vi "BAR0469_MainProject2.vi"() -> ()   [LabVIEW 2021]
panel:
  out "Vypoctena Fmez":dbl caption="Vypoctena Fmez (Hz)"
  out "Aktuální amplituda (V)":dbl
  out "A/f charakteristika":cluster{dbl[], dbl[]}(graph)
  in  "liner/log":bool
  in  "Typ filtru":string
  in  "Krok":dbl min=0.0 max=10000.0
  in  "Aproximace":string
  in  "Amplituda (V)":dbl min=0.0 max=10.0
  out "Aktuální frekvence (Hz)":dbl
  in  "volt/dB":bool
  in  "Vysoká frekvence (Hz)":dbl min=0.0 max=10000.0
  in  "Nízká frekvence (Hz)":dbl min=0.0 max=10000.0
  in  "Øád":i8 min=0 max=6
  in  "fmin (Hz)":dbl min=0.0 max=10000.0
  in  "fmax (Hz)":dbl min=0.0 max=1000.0
  in  "Username":string caption="Jméno Uživatele"
  in  "Stop":bool caption="OK Button"
  in  "Save button":bool caption="OK Button"
  in  "Load":bool caption="OK Button"
  in  "Reincialization Button":bool caption="OK Button"
  in  "Start Button":bool caption="OK Button"
  out "Datum a èas mìøení":string
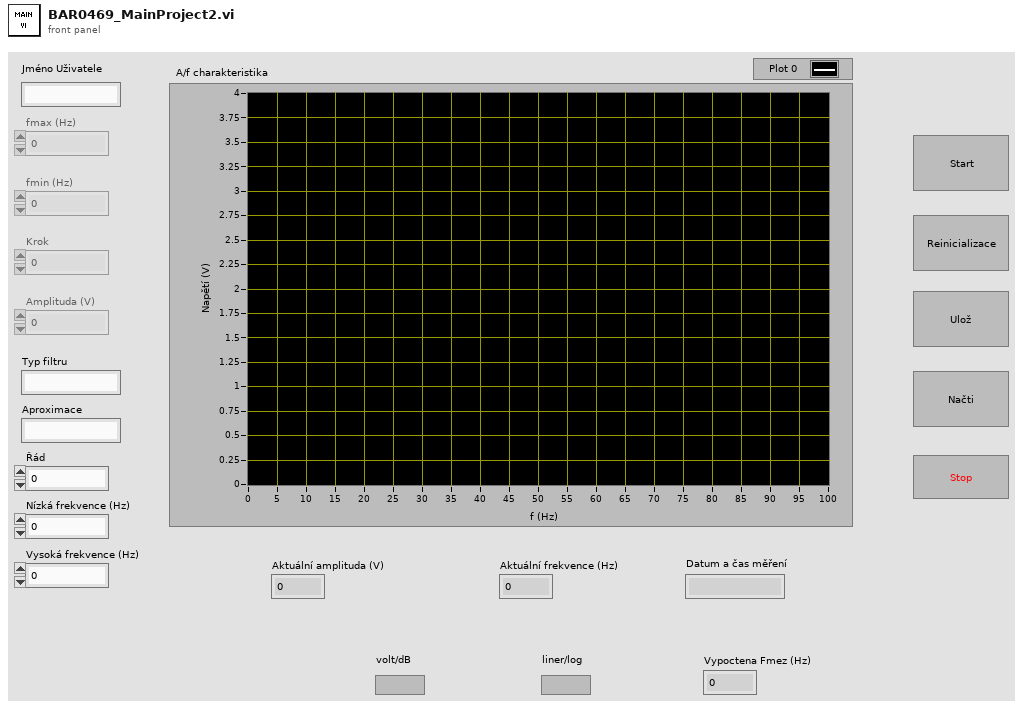
[diagram p1: front panel]
types:
  T1 = enum8{"Enabled", "Disabled", "Disabled and Grayed Out"}
  T2 = cluster{"Frequency (Hz)":dbl[], "Pøenos (dB)":dbl[]}
  T3 = cluster{"Frequency (Hz)":dbl[], "Amplitude (V)":dbl[]}
  T4 = cluster{"String from file":string, "String from file":string, "String from file":string, "String from file":string, "String from file":string, "String from file":string, "String from file":string, "String from file":string, "String from file":string, "String from file":string, "String from file":string}
  T5 = cluster{"Frequency (Hz)":dbl[], "Amplitude (V)":dbl[], "Pøenos (dB)":dbl[]}
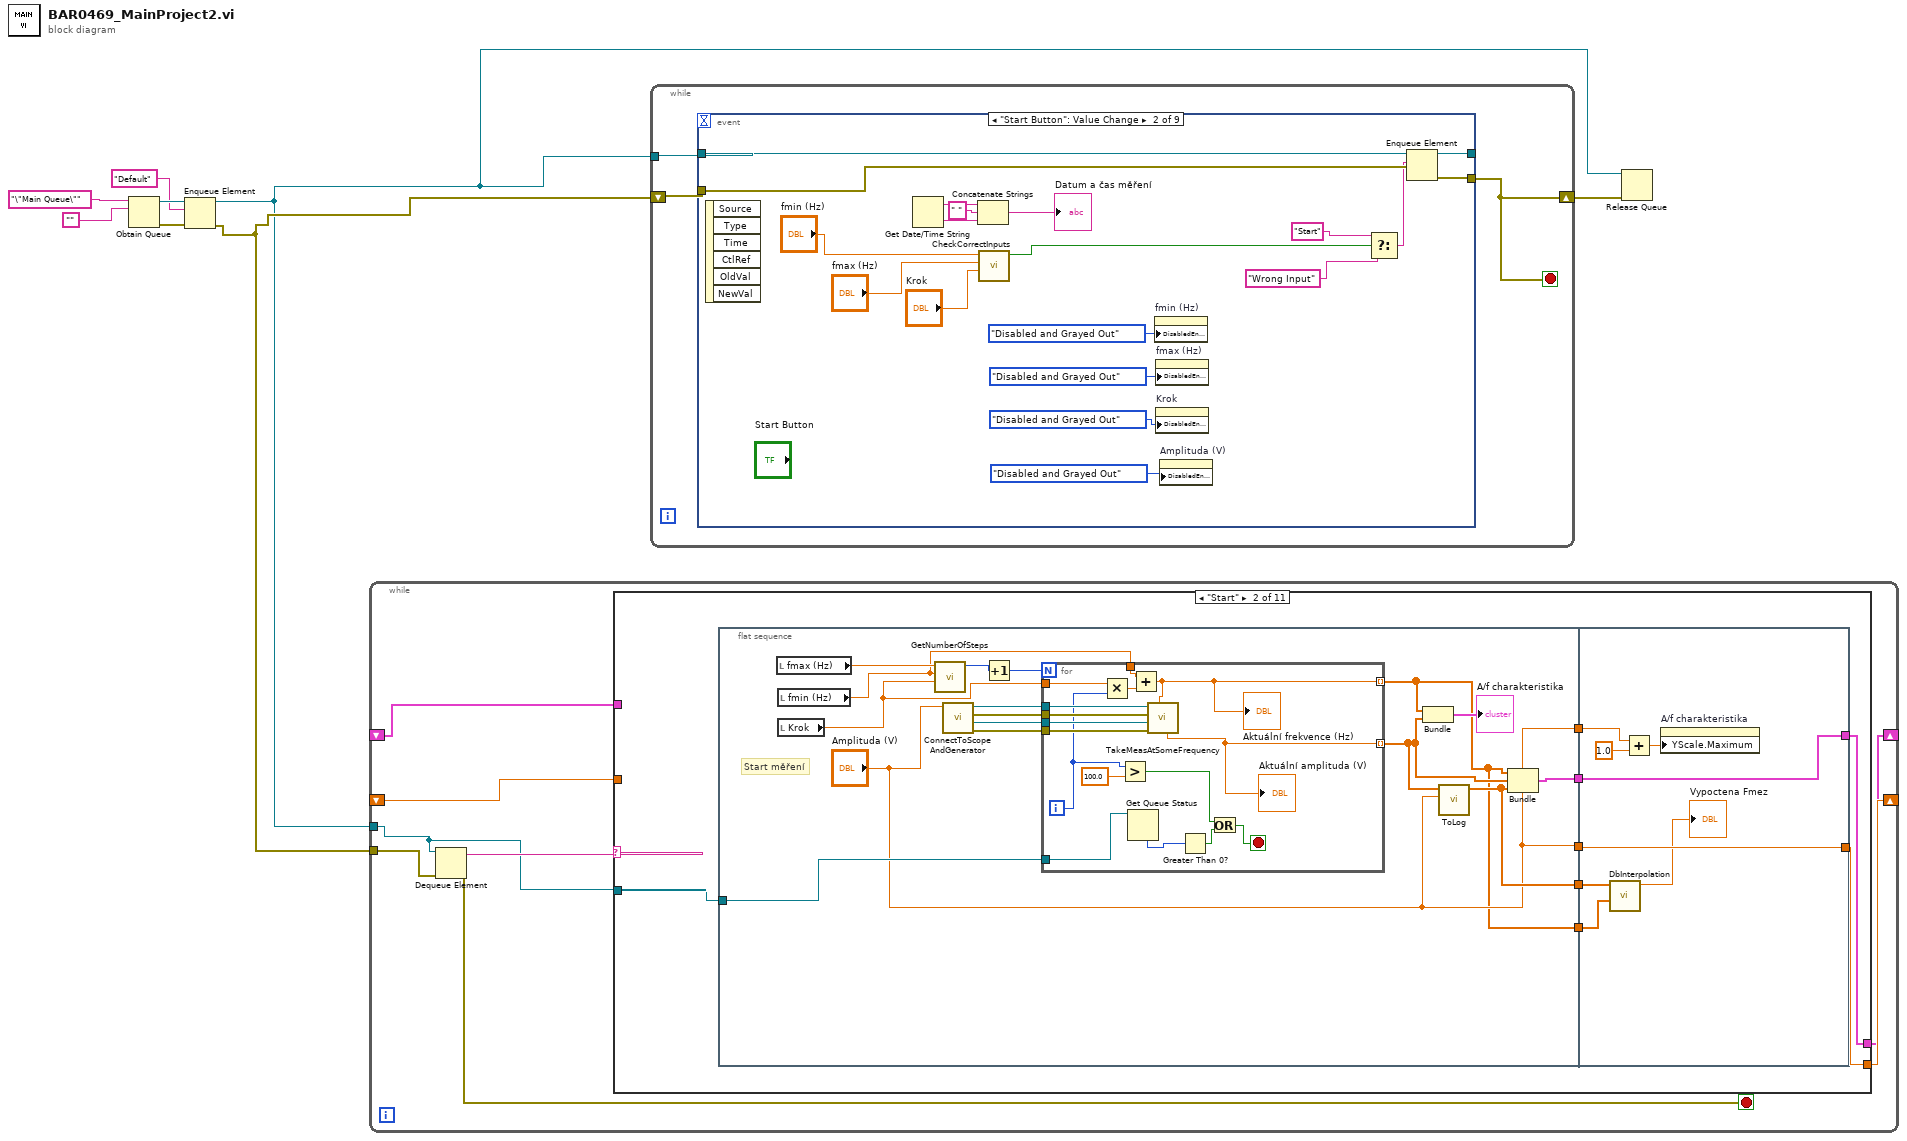
[diagram p0: block diagram]
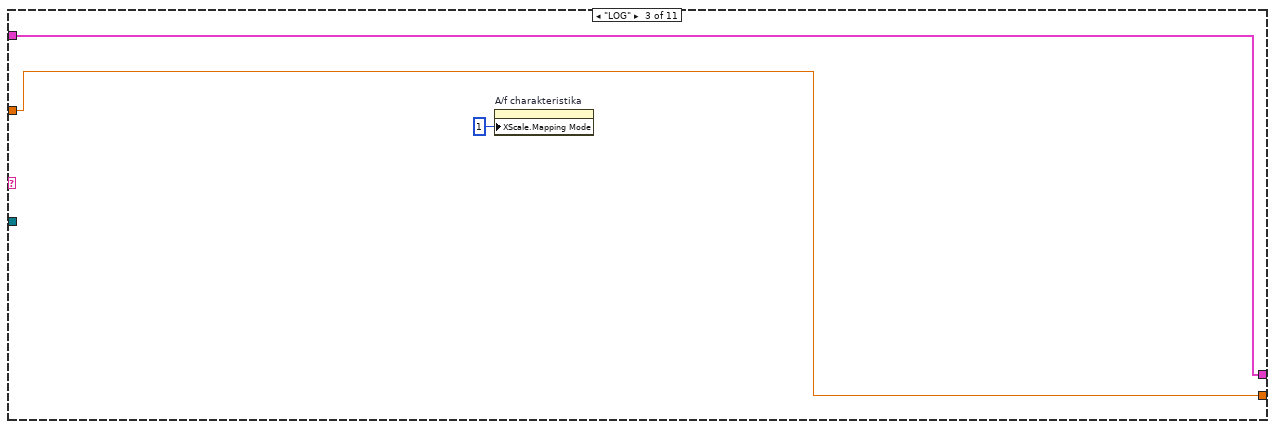
[diagram p3: hidden frame]
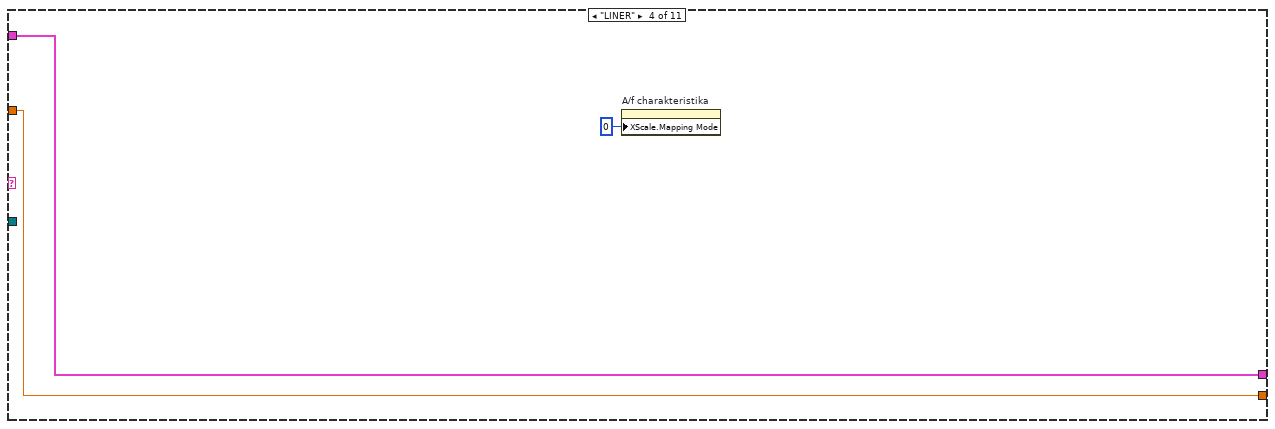
[diagram p4: hidden frame]
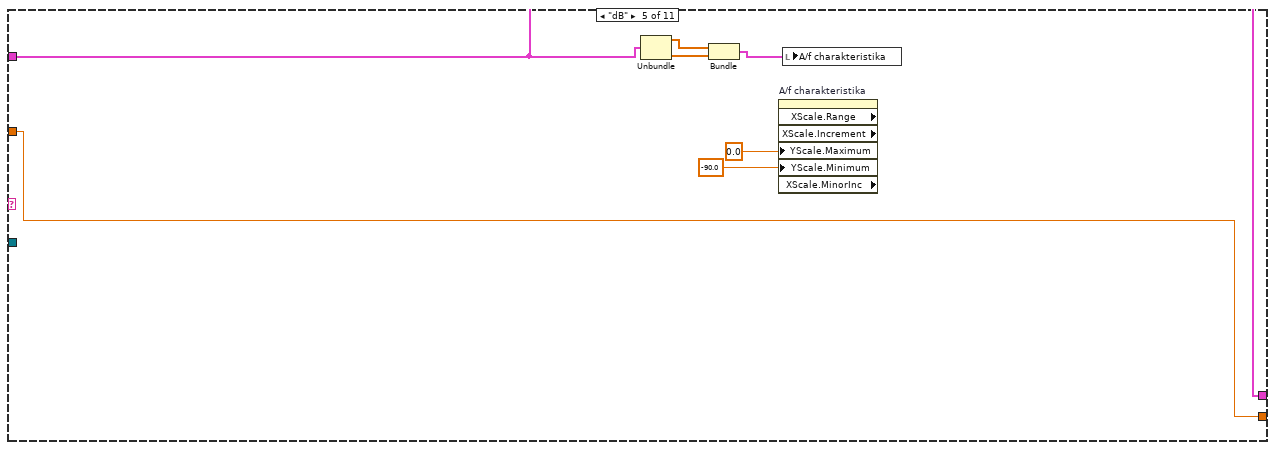
[diagram p5: hidden frame]
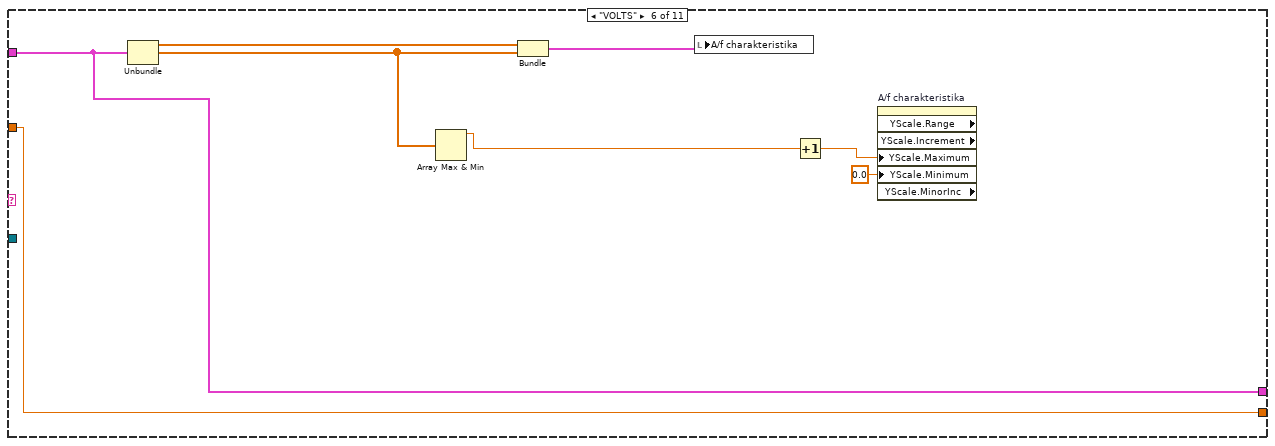
[diagram p6: hidden frame]
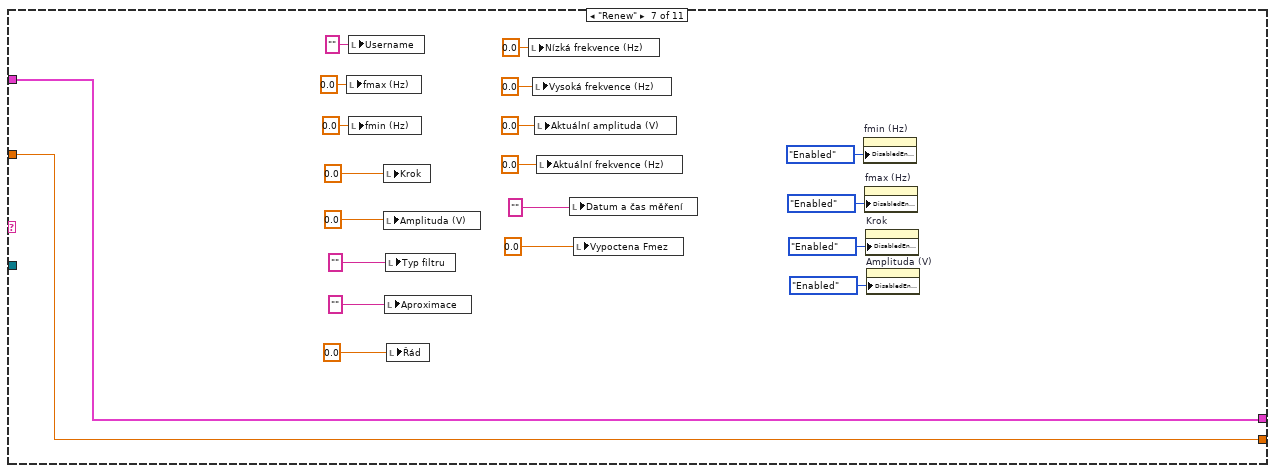
[diagram p7: hidden frame]
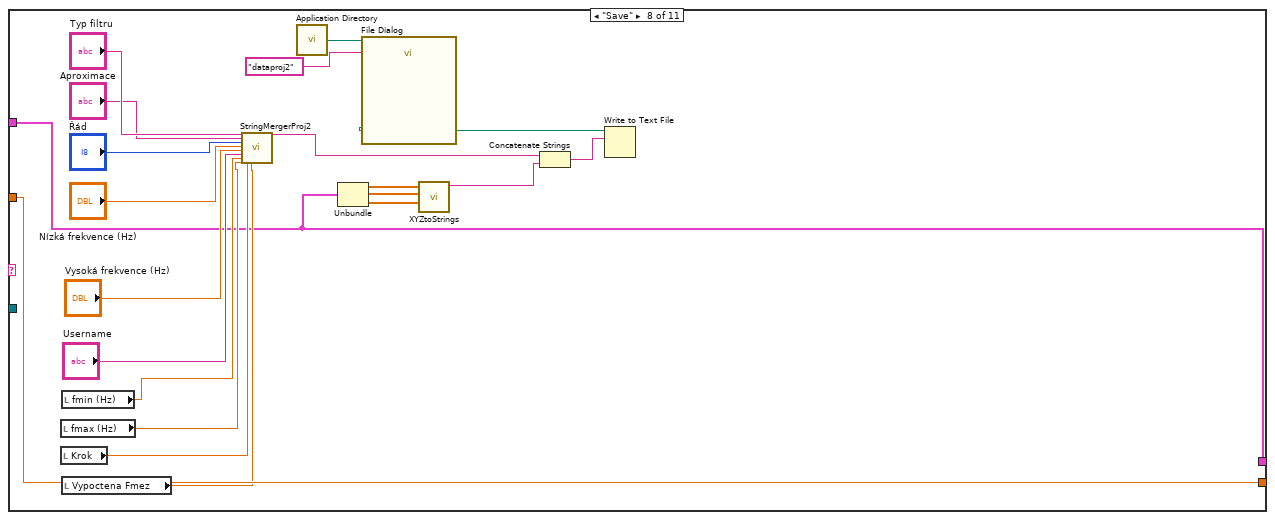
[diagram p8: hidden frame]
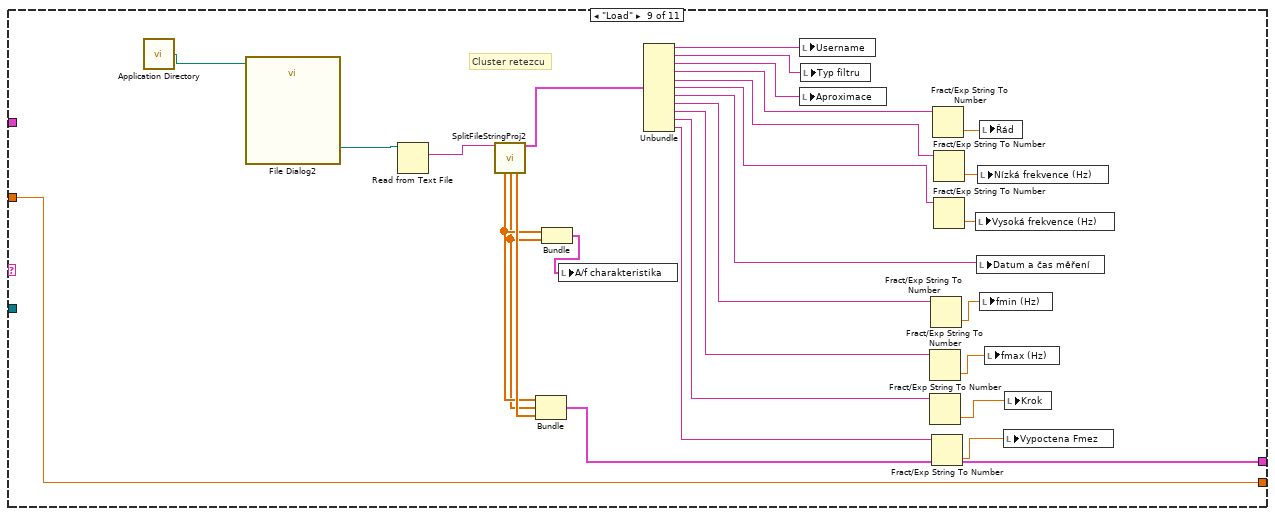
[diagram p9: hidden frame]
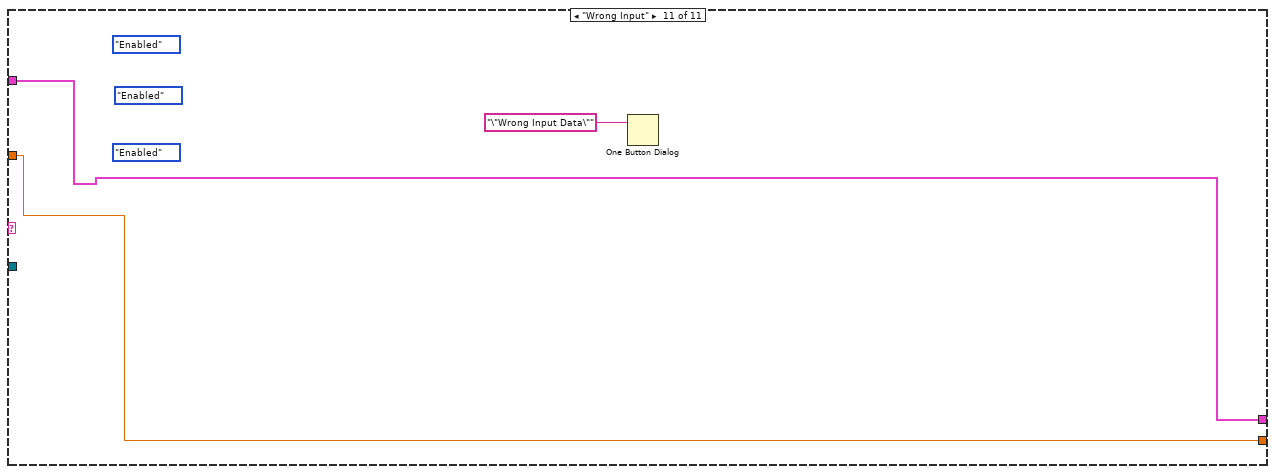
[diagram p11: hidden frame]
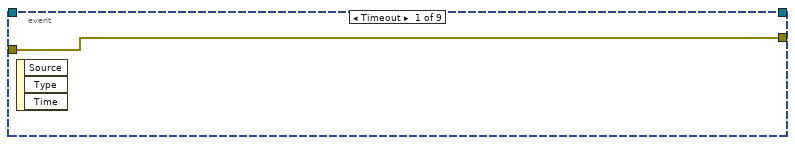
[diagram p12: hidden frame]
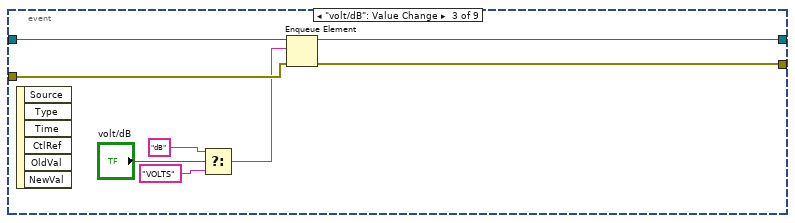
[diagram p13: hidden frame]
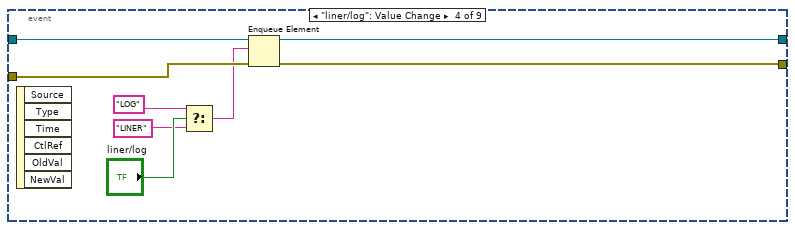
[diagram p14: hidden frame]
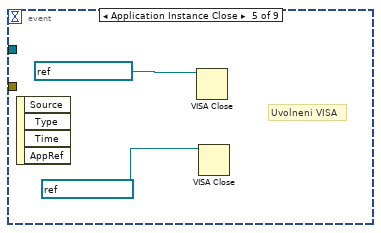
[diagram p15: hidden frame]
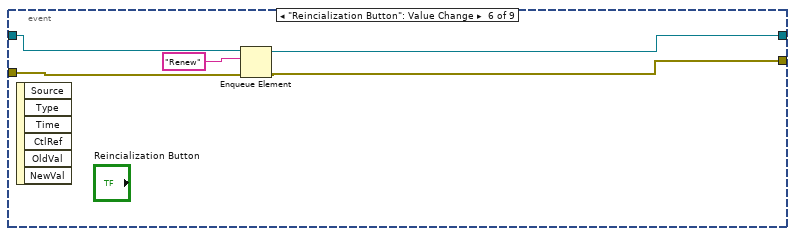
[diagram p16: hidden frame]
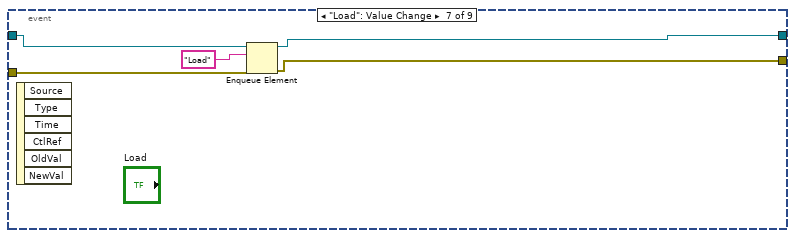
[diagram p17: hidden frame]
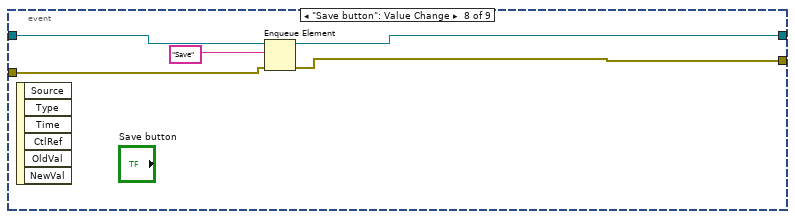
[diagram p18: hidden frame]
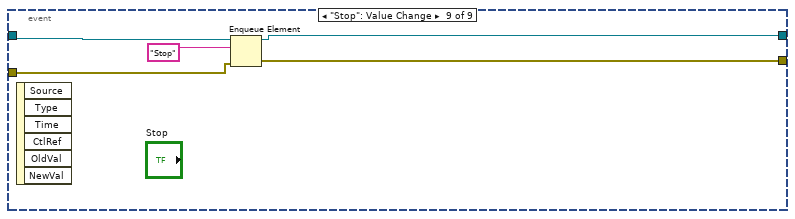
[diagram p19: hidden frame]
diagram:
  n1 = Obtain Queue(name (unnamed)="\"Main Queue\"", element data type="") -> (queue out=w6:refnum<queue>, error out=w5:errorcluster)  [unwired: 3 in, 1 out]
  n2 = Enqueue Element(queue=w6, element="Default", error in (no error)=w5) -> (queue out=w3:refnum<queue>, error out=w4:errorcluster)  [unwired: 1 in, 1 out]
  n3 = while {
    tunnel: w3 -> [w13]
    tunnel: w4 -> [w16]
    shift-right: [w12] -> _
    shift-left: _ -> [w11]
    shift-right: [w10] -> _
    shift-left: _ -> [w9]
    stop <- w15 stop-if-true
    n4 = Dequeue Element(queue=w13, error in (no error)=w16) -> (element=w14:string, error out=w15:errorcluster)  [unwired: 1 in, 2 out]
    n5 = case shown="\"Start\"" w14 {
      tunnel: w13 -> [_ w26 _ _ _ _ _ _ _ _ _]
      tunnel: [w18 w23 w67 w71 w77 w80 w107 w128 w156 w158 w160] -> w12
      tunnel: w11 -> [w18 _ w67 w71 w77 w80 w107 w128 w156 w158 w160]
      tunnel: [w17 w22 w68 w72 w73 w83 w106 w114 w132 w157 w159] -> w10
      tunnel: w9 -> [w17 _ w68 w72 w73 w83 w106 w114 _ w157 w159]
      frame "Default", Default {
      }
      frame "Start" {
        n6 = flat-sequence {
          tunnel: w26 -> [w35]
          tunnel: ["Amplituda (V)"] -> w25
          tunnel: ["Amplituda (V)"] -> w24
          tunnel: [w32] -> w21
          tunnel: [w31] -> w20
          tunnel: [w29] -> w19
          tunnel: w25 -> [w64]
          tunnel: w24 -> [w63]
          tunnel: [w63] -> w23
          tunnel: [w62] -> w22
          tunnel: w21 -> [w62]
          tunnel: w20 -> [w61]
          tunnel: w19 -> [w60]
          frame #0 {
            # "Start mìøení"
            n7 = local read "fmax (Hz)"() -> (w38:dbl)
            n8 = local read "fmin (Hz)"() -> (w36:dbl)
            n9 = local read "Krok"() -> (w37:dbl)
            n10 = call "GetNumberOfSteps.vi"("Step"=w37, "Min"=w36, "Max"=w38) -> ("unsigned 64bit integer"=w28:u64)  [unwired: 8 in]
            n11 = call "ConnectToScopeAndGenerator.vi"("Input Number"="Amplituda (V)") -> ("GEN error out"=w39:errorcluster, "GEN resource output"=w40:refnum<visa-resource-name>, "OSC error out"=w41:errorcluster, "OSC Reference"=w42:refnum<visa-resource-name>)  [unwired: 7 in]
            n12 = Increment(x=w28) -> (x+1=w27:u64)
            n13 = for {
              N: w27 -> [_]
              tunnel: w42 -> [w58]
              tunnel: w41 -> [w57]
              tunnel: w40 -> [w56]
              tunnel: w39 -> [w55]
              tunnel: [w54] -> w33 mode=indexing
              tunnel: w37 -> [w53]
              tunnel: w36 -> [w51]
              tunnel: [w48] -> w29 mode=indexing
              tunnel: w35 -> [w49]
              i -> [w46]
              stop <- w44 stop-if-true
              n14 = Multiply(x=w53, y=w46) -> (x*y=w52:dbl)
              n15 = Greater?(x=w46, y=100.0) -> (0:w43:bool)
              n16 = Get Queue Status(queue=w49) -> (# elements in queue=w50:i32)  [unwired: 2 in, 7 out]
              n17 = Add(x=w51, y=w52) -> (x+y=w48:dbl)
              "Aktuální frekvence (Hz)" <- w48
              n18 = call "TakeMeasAtSomeFrequency.vi"("Generator Frequency"=w48, "GEN error"=w55, "GEN VISA"=w56, "Scope Error"=w57, "Scope VISA"=w58) -> ("max value"=w54:dbl)  [unwired: 1 in, 5 out]
              "Aktuální amplituda (V)" <- w54
              n19 = Greater Than 0?(x=w50) -> (x > 0?=w45:bool)
              n20 = Or(x=w43, y=w45) -> (x .or. y?=w44:bool)
            }
            n21 = Bundle(w29, w33) -> (→"A/f charakteristika":cluster{dbl[], dbl[]})  [unwired: 1 in]
            n22 = call "ToLog.vi"("Amplituda"="Amplituda (V)", "Pole vystupniho napeti"=w33) -> ("Napeti log"=w31:dbl[])  [unwired: 9 in]
            n23 = Bundle(w29, w33, "Napeti log"=w31) -> (w32:cluster{dbl[], dbl[], "Napeti log":dbl[]})  [unwired: 1 in]
          }
          frame #1 {
            n24 = call "DbInterpolation.vi"("Frequency"=w60, "Transfers"=w61) -> ("interpolated val"=→"Vypoctena Fmez":dbl)  [unwired: 9 in]
            n25 = Add(x=w64, y=1.0) -> (x+y=w66:dbl)
            n26 = property on="A/f charakteristika" class="XYGraph (strict)"("YScale.Maximum"=w66) -> ()  [unwired: 2 in, 2 out]
          }
        }
      }
      frame "LOG" {
        n27 = property on="A/f charakteristika" class="XYGraph (strict)"("XScale.Mapping Mode"=u8 1 ("X Scale.Mapping Mode")) -> ()  [unwired: 2 in, 2 out]
      }
      frame "LINER" {
        n28 = property on="A/f charakteristika" class="XYGraph (strict)"("XScale.Mapping Mode"=u8 0 ("Y Scale.Mapping Mode")) -> ()  [unwired: 2 in, 2 out]
      }
      frame "dB" {
        n29 = Unbundle(w73) -> ("Frequency (Hz)"=w76:dbl[], "Pøenos (dB)"=w75:dbl[])  [unwired: 1 out]
        n30 = Bundle("Frequency (Hz)"=w76, "Pøenos (dB)"=w75) -> (w74:T2)  [unwired: 1 in]
        n31 = property on="A/f charakteristika" class="XYGraph (strict)" props=["XScale", "Range", "XScale", "Increment", "YScale", "Maximum", "YScale", "Minimum", "XScale", "MinorInc"]("YScale.Maximum"=0.0 ("X Scale.Range:Maximum"), "YScale.Minimum"=-90.0 ("X Scale.Range:Minimum")) -> ()  [unwired: 2 in, 5 out]
        n32 = local write "A/f charakteristika"(w74) -> ()
      }
      frame "VOLTS" {
        n33 = Unbundle(w83) -> ("Frequency (Hz)"=w85:dbl[], "Amplitude (V)"=w82:dbl[])  [unwired: 1 out]
        n34 = Array Max & Min(array=w82) -> (max value=w81:dbl)  [unwired: 3 out]
        n35 = Bundle("Frequency (Hz)"=w85, "Amplitude (V)"=w82) -> (w84:T3)  [unwired: 1 in]
        n36 = local write "A/f charakteristika"(w84) -> ()
        n37 = Increment(x=w81) -> (x+1=w86:dbl)
        n38 = property on="A/f charakteristika" class="XYGraph (strict)" props=["YScale", "Range", "YScale", "Increment", "YScale", "Maximum", "YScale", "Minimum", "YScale", "MinorInc"]("YScale.Maximum"=w86, "YScale.Minimum"=0.0 ("Y Scale.Range:Minimum")) -> ()  [unwired: 2 in, 5 out]
      }
      frame "Renew" {
        n39 = local write "fmax (Hz)"(0.0 ("fmax (Hz)")) -> ()
        n40 = local write "Username"("" ("Username")) -> ()
        n41 = local write "fmin (Hz)"(0.0 ("fmin (Hz)")) -> ()
        n42 = local write "Krok"(0.0 ("Krok")) -> ()
        n43 = local write "Amplituda (V)"(0.0 ("Amplituda (V)")) -> ()
        n44 = local write "Aproximace"("" ("Aproximace")) -> ()
        n45 = local write "Typ filtru"("" ("Typ filtru")) -> ()
        n46 = local write "Øád"(0.0 ("Øád")) -> ()
        n47 = local write "Nízká frekvence (Hz)"(0.0 ("Nízká frekvence (Hz)")) -> ()
        n48 = local write "Vysoká frekvence (Hz)"(0.0 ("Vysoká frekvence (Hz)")) -> ()
        n49 = local write "Aktuální amplituda (V)"(0.0 ("Aktuální amplituda (V)")) -> ()
        n50 = local write "Aktuální frekvence (Hz)"(0.0 ("Aktuální frekvence (Hz)")) -> ()
        n51 = local write "Datum a èas mìøení"("" ("Datum a èas mìøení")) -> ()
        n52 = local write "Vypoctena Fmez"(0.0 ("Vypoctena Fmez")) -> ()
        n53 = property on="fmin (Hz)" class="DigNum (strict)"("DisabledEnum"=T1."Enabled" ("Disabled")) -> ()  [unwired: 2 in, 2 out]
        n54 = property on="fmax (Hz)" class="DigNum (strict)"("DisabledEnum"=T1."Enabled" ("Disabled")) -> ()  [unwired: 2 in, 2 out]
        n55 = property on="Krok" class="DigNum (strict)"("DisabledEnum"=T1."Enabled" ("Disabled")) -> ()  [unwired: 2 in, 2 out]
        n56 = property on="Amplituda (V)" class="DigNum (strict)"("DisabledEnum"=T1."Enabled" ("Disabled")) -> ()  [unwired: 2 in, 2 out]
      }
      frame "Save" {
        n57 = local read "fmax (Hz)"() -> (w118:dbl)
        n58 = local read "Krok"() -> (w117:dbl)
        n59 = local read "fmin (Hz)"() -> (w119:dbl)
        n60 = local read "Vypoctena Fmez"() -> (w116:dbl)
        n61 = call "StringMergerProj2.vi"("FilterType"="Typ filtru", "Aproximace"="Aproximace", "Rad"="Øád", "Nizka frekvence"="Nízká frekvence (Hz)", "Vysoka frekvence"="Vysoká frekvence (Hz)", "Username"="Username", "Min Frequency"=w119, "Max Frequency"=w118, "Step"=w117, "Fmez"=w116) -> ("Output string"=w109:string)  [unwired: 17 in]
        n62 = call <vilib>:"Application Directory.vi"() -> ("Application Directory"=w127:path)
        n63 = Unbundle(w114) -> ("Frequency (Hz)"=w113:dbl[], "Amplitude (V)"=w112:dbl[], "Pøenos (dB)"=w111:dbl[])
        n64 = call "File Dialog"("start path"=w127, "default name"="dataproj2") -> ("selected path"=w115:path)  [unwired: 10 in, 3 out]
        n65 = call "XYZtoStrings.vi"("Pøenos (dB)"=w111, "Amplituda (V)"=w112, "Frekvence (Hz)"=w113) -> ("concatenated string"=w108:string)  [unwired: 8 in]
        n66 = Concatenate Strings(w109, w108) -> (w110:string)
        n67 = Write to Text File(file (use dialog)=w115, text=w110) -> ()  [unwired: 2 in, 3 out]
      }
      frame "Load" {
        # "Cluster retezcu"
        n68 = call <vilib>:"Application Directory.vi"() -> ("Application Directory"=w155:path)
        n69 = call "File Dialog2"("start path"=w155) -> ("selected path"=w154:path)  [unwired: 11 in, 3 out]
        n70 = Read from Text File(file (use dialog)=w154) -> (text=w153:string)  [unwired: 3 in, 3 out]
        n71 = call "SplitFileStringProj2.vi"("String from file"=w153) -> ("output cluster"=w152:T4, "Frequency (Hz)"=w131:dbl[], "Amplitude (V)"=w130:dbl[], "Pøenos (dB)"=w133:dbl[])  [unwired: 11 in]
        n72 = Bundle("Frequency (Hz)"=w131, "Amplitude (V)"=w130, "Pøenos (dB)"=w133) -> (w132:T5)  [unwired: 1 in]
        n73 = Bundle("Frequency (Hz)"=w131, "Amplitude (V)"=w130) -> (w129:T3)  [unwired: 1 in]
        n74 = local write "A/f charakteristika"(w129) -> ()
        n75 = Unbundle(w152) -> ("String from file"=w151:string, "String from file"=w150:string, "String from file"=w149:string, "String from file"=w147:string, "String from file"=w145:string, "String from file"=w144:string, "String from file"=w142:string, "String from file"=w140:string, "String from file"=w138:string, "String from file"=w137:string, "String from file"=w135:string)
        n76 = local write "Username"(w151) -> ()
        n77 = local write "Aproximace"(w149) -> ()
        n78 = local write "Typ filtru"(w150) -> ()
        n79 = Fract/Exp String To Number(string=w138) -> (number=w139:dbl)  [unwired: 3 in, 1 out]
        n80 = Fract/Exp String To Number(string=w137) -> (number=w136:dbl)  [unwired: 3 in, 1 out]
        n81 = Fract/Exp String To Number(string=w140) -> (number=w141:dbl)  [unwired: 3 in, 1 out]
        n82 = Fract/Exp String To Number(string=w135) -> (number=w134:dbl)  [unwired: 3 in, 1 out]
        n83 = Fract/Exp String To Number(string=w147) -> (number=w148:dbl)  [unwired: 3 in, 1 out]
        n84 = Fract/Exp String To Number(string=w145) -> (number=w146:dbl)  [unwired: 3 in, 1 out]
        n85 = Fract/Exp String To Number(string=w144) -> (number=w143:dbl)  [unwired: 3 in, 1 out]
        n86 = local write "Vysoká frekvence (Hz)"(w143) -> ()
        n87 = local write "Datum a èas mìøení"(w142) -> ()
        n88 = local write "Nízká frekvence (Hz)"(w146) -> ()
        n89 = local write "Øád"(w148) -> ()
        n90 = local write "fmin (Hz)"(w141) -> ()
        n91 = local write "fmax (Hz)"(w139) -> ()
        n92 = local write "Vypoctena Fmez"(w134) -> ()
        n93 = local write "Krok"(w136) -> ()
      }
      frame "Stop" {
      }
      frame "Wrong Input" {
        (unwired) T1."Enabled" ("Disabled")
        (unwired) T1."Enabled" ("Disabled")
        (unwired) T1."Enabled" ("Disabled")
        n94 = One Button Dialog(message="\"Wrong Input Data\"") -> ()  [unwired: 1 in, 1 out]
      }
    }
  }
  n95 = while {
    shift-right: [w162] -> w7
    shift-left: w4 -> [w164]
    tunnel: w3 -> [w163]
    stop <- w162 stop-if-true
    n96 = event shown="[1] \"Start Button\": Value Change" {
      selector: _ -> [_ _ _ _ _ _ _ _ _]
      dyn-events: _ -> [_ _ _ _ _ _ _ _ _]
      timeout: _ -> [_ _ _ _ _ _ _ _ _]
      tunnel: w164 -> [w165 w184 w189 w198 _ w206 w209 w217 w222]
      tunnel: [w165 w183 w188 w197 _ w204 w210 w214 w219] -> w162
      tunnel: w163 -> [_ w182 w192 w200 _ w207 w212 w216 w221]
      tunnel: [_ w181 w191 w199 _ w205 w211 w215 w220] -> _
      event Timeout {
        n97 = event-data() -> ()  [unwired: 1 in, 3 out]
      }
      event "Start Button": Value Change {
        n98 = event-data() -> ()  [unwired: 1 in, 6 out]
        n99 = Get Date/Time String() -> (date string=w177:string, time string=w174:string)  [unwired: 3 in]
        n100 = Concatenate Strings(w177, " " ("string"), w174) -> (→"Datum a èas mìøení":string)
        n101 = call "CheckCorrectInputs.vi"("Step"="Krok", "Max"="fmax (Hz)", "Min"="fmin (Hz)") -> ("x .or. y?"=w170:bool)  [unwired: 8 in]
        n102 = property on="fmin (Hz)" class="DigNum (strict)"("DisabledEnum"=T1."Disabled and Grayed Out" ("Disabled")) -> ()  [unwired: 2 in, 2 out]
        n103 = property on="fmax (Hz)" class="DigNum (strict)"("DisabledEnum"=T1."Disabled and Grayed Out" ("Disabled")) -> ()  [unwired: 2 in, 2 out]
        n104 = property on="Krok" class="DigNum (strict)"("DisabledEnum"=T1."Disabled and Grayed Out" ("Disabled")) -> ()  [unwired: 2 in, 2 out]
        n105 = property on="Amplituda (V)" class="DigNum (strict)"("DisabledEnum"=T1."Disabled and Grayed Out" ("Disabled")) -> ()  [unwired: 2 in, 2 out]
        n106 = Select(t="Start", s=w170, f="Wrong Input") -> (s? t:f=w180:string)
        n107 = Enqueue Element(queue=w182, element=w180, error in (no error)=w184) -> (queue out=w181:refnum<queue>, error out=w183:errorcluster)  [unwired: 1 in, 1 out]
      }
      event "volt/dB": Value Change {
        n108 = event-data() -> ()  [unwired: 1 in, 6 out]
        n109 = Select(t="dB", s="volt/dB", f="VOLTS") -> (s? t:f=w185:string)
        n110 = Enqueue Element(queue=w192, element=w185, error in (no error)=w189) -> (queue out=w191:refnum<queue>, error out=w188:errorcluster)  [unwired: 1 in, 1 out]
      }
      event "liner/log": Value Change {
        n111 = event-data() -> ()  [unwired: 1 in, 6 out]
        n112 = Select(t="LOG", s="liner/log", f="LINER") -> (s? t:f=w196:string)
        n113 = Enqueue Element(queue=w200, element=w196, error in (no error)=w198) -> (queue out=w199:refnum<queue>, error out=w197:errorcluster)  [unwired: 1 in, 1 out]
      }
      event Application Instance Close {
        # "Uvolneni VISA"
        n114 = event-data() -> ()  [unwired: 1 in, 4 out]
        n115 = VISA Close(VISA resource name=refnum<visa-resource-name> "FG_Simulator") -> ()  [unwired: 1 in, 1 out]
        n116 = VISA Close(VISA resource name=refnum<visa-resource-name> "Osciloscope") -> ()  [unwired: 1 in, 1 out]
      }
      event "Reincialization Button": Value Change {
        n117 = event-data() -> ()  [unwired: 1 in, 6 out]
        n118 = Enqueue Element(queue=w207, element="Renew", error in (no error)=w206) -> (queue out=w205:refnum<queue>, error out=w204:errorcluster)  [unwired: 1 in, 1 out]
      }
      event "Load": Value Change {
        n119 = event-data() -> ()  [unwired: 1 in, 6 out]
        n120 = Enqueue Element(queue=w212, element="Load", error in (no error)=w209) -> (queue out=w211:refnum<queue>, error out=w210:errorcluster)  [unwired: 1 in, 1 out]
      }
      event "Save button": Value Change {
        n121 = event-data() -> ()  [unwired: 1 in, 6 out]
        n122 = Enqueue Element(queue=w216, element="Save", error in (no error)=w217) -> (queue out=w215:refnum<queue>, error out=w214:errorcluster)  [unwired: 1 in, 1 out]
      }
      event "Stop": Value Change {
        n123 = event-data() -> ()  [unwired: 1 in, 6 out]
        n124 = Enqueue Element(queue=w221, element="Stop", error in (no error)=w222) -> (queue out=w220:refnum<queue>, error out=w219:errorcluster)  [unwired: 1 in, 1 out]
      }
    }
  }
  n125 = Release Queue(queue=w3, error in (no error)=w7) -> ()  [unwired: 1 in, 3 out]
